vi "Periodic Tasks Curtis.vi"(8 "error in":errorcluster) -> ()   [LabVIEW 2016]
doc: "This VI runs in parallel to other tasks. It can contain as many user-defined periodic loops as you need. These can carry out PID or other sorts of timed response."
uses:
  <userlib>/836-libraries/Drive/Drive_Code/Drive_Code_Support/Drive_Code_PID_Bundle.ctl
  <vilib>/Platform/TimedLoop/XDataNode/timing_clust.ctl
  <vilib>/Platform/TimedLoop/XDataNode/nitl_modes.ctl
  <vilib>/Platform/TimedLoop/XDataNode/wakeup.ctl
  <vilib>/Rock Robotics/WPI/RobotDrive/WPI_RobotDriveDevRef.ctl
  <vilib>/Rock Robotics/WPI/MotorControl/WPI_MotorControlDeviceRef.ctl
  <vilib>/Rock Robotics/WPI/MotorControl/WPI_MotorControlType.ctl
  <vilib>/Rock Robotics/SystemInterfaces/DIO/FPGA_DIOPWMChannel.ctl
  <vilib>/Rock Robotics/WPI/PWM/WPI_PWMDeadband.ctl
  <vilib>/Rock Robotics/WPI/ThirdParty/CanMotor/TalonSRX/WPI_CANTalonSRX_APIControlMode.ctl
  <vilib>/Rock Robotics/WPI/Utilities/WPI_GetSetVariantRefNum.vi
  <vilib>/addons/control/pid/pid.llb/PID (DBL).vi
  <vilib>/platform/TimedLoop/XDataNode/XDataNode.xnode
  <vilib>/Platform/TimedLoop/XDataNode/XDNodeRunTimeDep.lvlib
  <vilib>/addons/control/pid/NI_PID_pid.lvlib
panel:
  in  "reset":bool
  in  "PID gains 2":T1={"proportional gain (Kc)"=0.025, "integral time (Ti, min)"=0.0, "derivative time (Td, min)"=0.01} {"derivative time (Td, min)" format="%.3f"; "integral time (Ti, min)" format="%.3f"; "proportional gain (Kc)" format="%.3f"}
  in  "Offset":dbl=20.0
  in  "Max Throttle":dbl=0.35
  in  "Negate":bool=TRUE
  in  "Follow Cam":bool=TRUE
  in  "PID Gains 2":T2={"Yaw, Driving Straight"={"proportional gain (Kc)"=0.08, "integral time (Ti, min)"=0.0, "derivative time (Td, min)"=0.0}, "Yaw, Holding Still"={"proportional gain (Kc)"=0.0, "integral time (Ti, min)"=0.0, "derivative time (Td, min)"=0.0}, "Distance, Driving Straight"={"proportional gain (Kc)"=0.0, "integral time (Ti, min)"=0.0, "derivative time (Td, min)"=0.0}, "Distance, Holding Still"={"proportional gain (Kc)"=0.0, "integral time (Ti, min)"=0.0, "derivative time (Td, min)"=0.0}}
  in  "reset":bool
  in  "PID Gains":T2
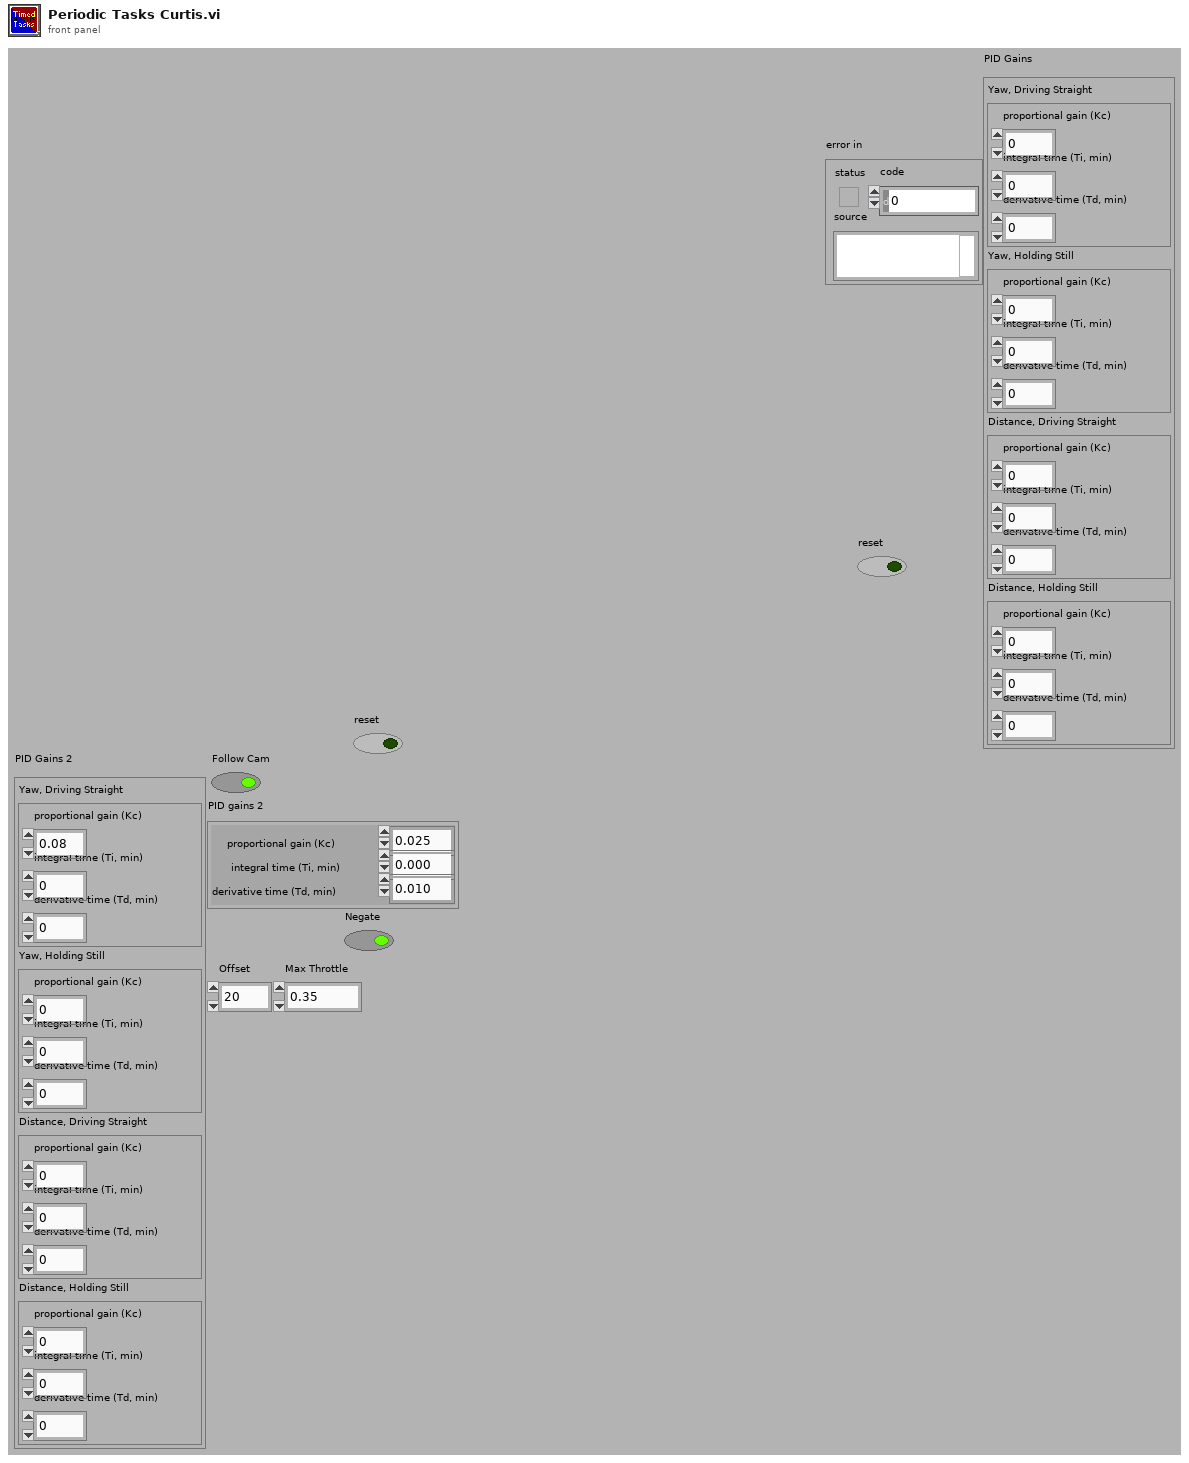
[diagram p1: front panel]
types:
  T1 = cluster{"proportional gain (Kc)":dbl, "integral time (Ti, min)":dbl, "derivative time (Td, min)":dbl}
  T2 = typedef "Drive_Code_PID_Bundle.ctl" = cluster{"Yaw, Driving Straight":cluster{"proportional gain (Kc)":dbl, "integral time (Ti, min)":dbl, "derivative time (Td, min)":dbl}, "Yaw, Holding Still":cluster{"proportional gain (Kc)":dbl, "integral time (Ti, min)":dbl, "derivative time (Td, min)":dbl}, "Distance, Driving Straight":cluster{"proportional gain (Kc)":dbl, "integral time (Ti, min)":dbl, "derivative time (Td, min)":dbl}, "Distance, Holding Still":cluster{"proportional gain (Kc)":dbl, "integral time (Ti, min)":dbl, "derivative time (Td, min)":dbl}}
  T3 = typedef "WPI_RobotDriveDevRef.ctl" = cluster{"DevStatus":errorcluster, "Motors[]":T4[], "Square Inputs":bool, "Max Output":dbl}
  T4 = typedef "WPI_MotorControlDeviceRef.ctl" = cluster{"DeviceStatus":errorcluster, "Type":T5, "PWM":cluster{"PWM Channel":T6, "DeadBand":T7}, "CAN":cluster{"Device Number":u8, "SetOutput VI Ref":variant, "GetOutput VI Ref":variant, "Enable VI Ref":variant, "Disable VI Ref":variant, "Data":variant}, "Invert":bool}
  T5 = typedef "WPI_MotorControlType.ctl" = enum16{"PWM", "CAN"}
  T6 = typedef "FPGA_DIOPWMChannel.ctl" = enum8{"PWM 0", "PWM 1", "PWM 2", "PWM 3", "PWM 4", "PWM 5", "PWM 6", "PWM 7", "PWM 8", "PWM 9", "PWM MXP 0", "PWM MXP 1", "PWM MXP 2", "PWM MXP 3", "PWM MXP 4", "PWM MXP 5", "PWM MXP 6", "PWM MXP 7", "PWM MXP 8", "PWM MXP 9", "Invalid"}
  T7 = typedef "WPI_PWMDeadband.ctl" = cluster{"Name":string, "maxPositivePwm":i32, "minPositivePwm":i32, "centerPwm":i32, "maxNegativePwm":i32, "minNegativePwm":i32, "angularRange":u16}
  T8 = typedef "WPI_JoystickDevRef.ctl" = cluster{"Device":T9}
  T9 = typedef "WPI_JoystickDeviceEnum.ctl" = enum16{"USB 0", "USB 1", "USB 2", "USB 3", "USB 4", "USB 5"}
  T10 = typedef "WPI_EncoderDevRef.ctl" = cluster{"DevStatus":errorcluster, "EncoderIndex":T11, "CounterIndex":T12, "DistancePerCount":dbl, "Decoding Type":T13}
  T11 = typedef "FPGA_EncoderIdx.ctl" = enum8{"Enc 0", "Enc 1", "Enc 2", "Enc 3", "Enc 4", "Enc 5", "Enc 6", "Enc 7", "Invalid"}
  T12 = typedef "FPGA_CounterCtrSystemIndex.ctl" = enum8{"Ctr 0", "Ctr 1", "Ctr 2", "Ctr 3", "Ctr 4", "Ctr 5", "Ctr 6", "Ctr 7", "Invalid"}
  T13 = typedef "WPI_EncoderType.ctl" = enum16{"1x", "2x", "4x"}
  T14 = cluster{"Yaw":dbl, "Roll":dbl, "Pitch":dbl, "Yaw Wind":dbl, "Roll Wind":dbl, "Pitch Wind":dbl}
  T15 = typedef "Drive_Code_Bundle.ctl" = cluster{"Sensor Data":T16, "Drive Command rt fifo":refnum<k33>, "Logging Data":refnum<k33>}
  T16 = typedef "Sensor_Cluster.ctl" = cluster{"Gyro Data":cluster{"Gyro RT FIFO":refnum<k33>, "Gyro Current":dbl, "Gyro Hold":dbl}, "Encoder Data":cluster{"Encoder RT FIFO":refnum<k33>, "Encoder Current":dbl, "Encoder Hold":dbl}, "Camera Data":cluster{"Camera RT FIFO":refnum<k33>, "Camera Current":T17}}
  T17 = typedef "Camera_Cluster.ctl" = cluster{" Angle":dbl, "Valid":bool}
  T18 = typedef "WPI_I2CDevRef.ctl" = cluster{"DevStatus":errorcluster, "Device Address":u8, "Handle":i32, "I2C Bus":T19}
  T19 = typedef "i2c_bus.ctl" = enum16{"I2C On-Board", "I2C MXP", "Invalid"}
  T20 = typedef "XDNodeRunTimeDep.lvlib/timing_clust.ctl" = cluster{"Expected End [f-1]":u64, "Actual End [f-1]":u64, "Finished Late? [f-1]":bool, "Expected End [i-1]":u64, "Actual End [i-1]":u64, "Finished Late? [i-1]":bool, "Expected Start [i]":u64, "Actual Start [i]":u64, "Expected Start [f]":u64, "Actual Start [f]":u64, "Source Name":string, "Structure Name":string, "Period":i64, "Deadline":i64, "Offset":i64, "Start":i64, "Priority":i32, "Timeout":i32, "Mode":T21, "Wakeup Reason":T22, "Error":errorcluster, "Source Type":string, "Secondary Source Type":string, "Global End Time":u64, "Global Start Time":u64, "Frame Duration":u64, "Iteration Duration":u64, "Assigned CPU":i32, "I/O Scan Engine Mode":u32}
  T21 = typedef "XDNodeRunTimeDep.lvlib/nitl_modes.ctl" = enum32{"No Change", "Process missed periods, maintain original phase", "Discard missed periods, maintain original phase", "Process missed periods, ignore original phase", "Discard missed periods, ignore original phase"}
  T22 = typedef "XDNodeRunTimeDep.lvlib/wakeup.ctl" = enum32{"Normal", "Aborted", "Asynchronous wakeup", "Timing source error", "Timed loop error", "Timeout"}
  T23 = typedef "WPI_CANTalonSRX_APIControlMode.ctl" = enum8{"Percent VBus", "Speed", "Position", "Slave", "Unchanged / Invalid", "Voltage Compensation", "Current", "Motion Profile", "Motion Magic"}
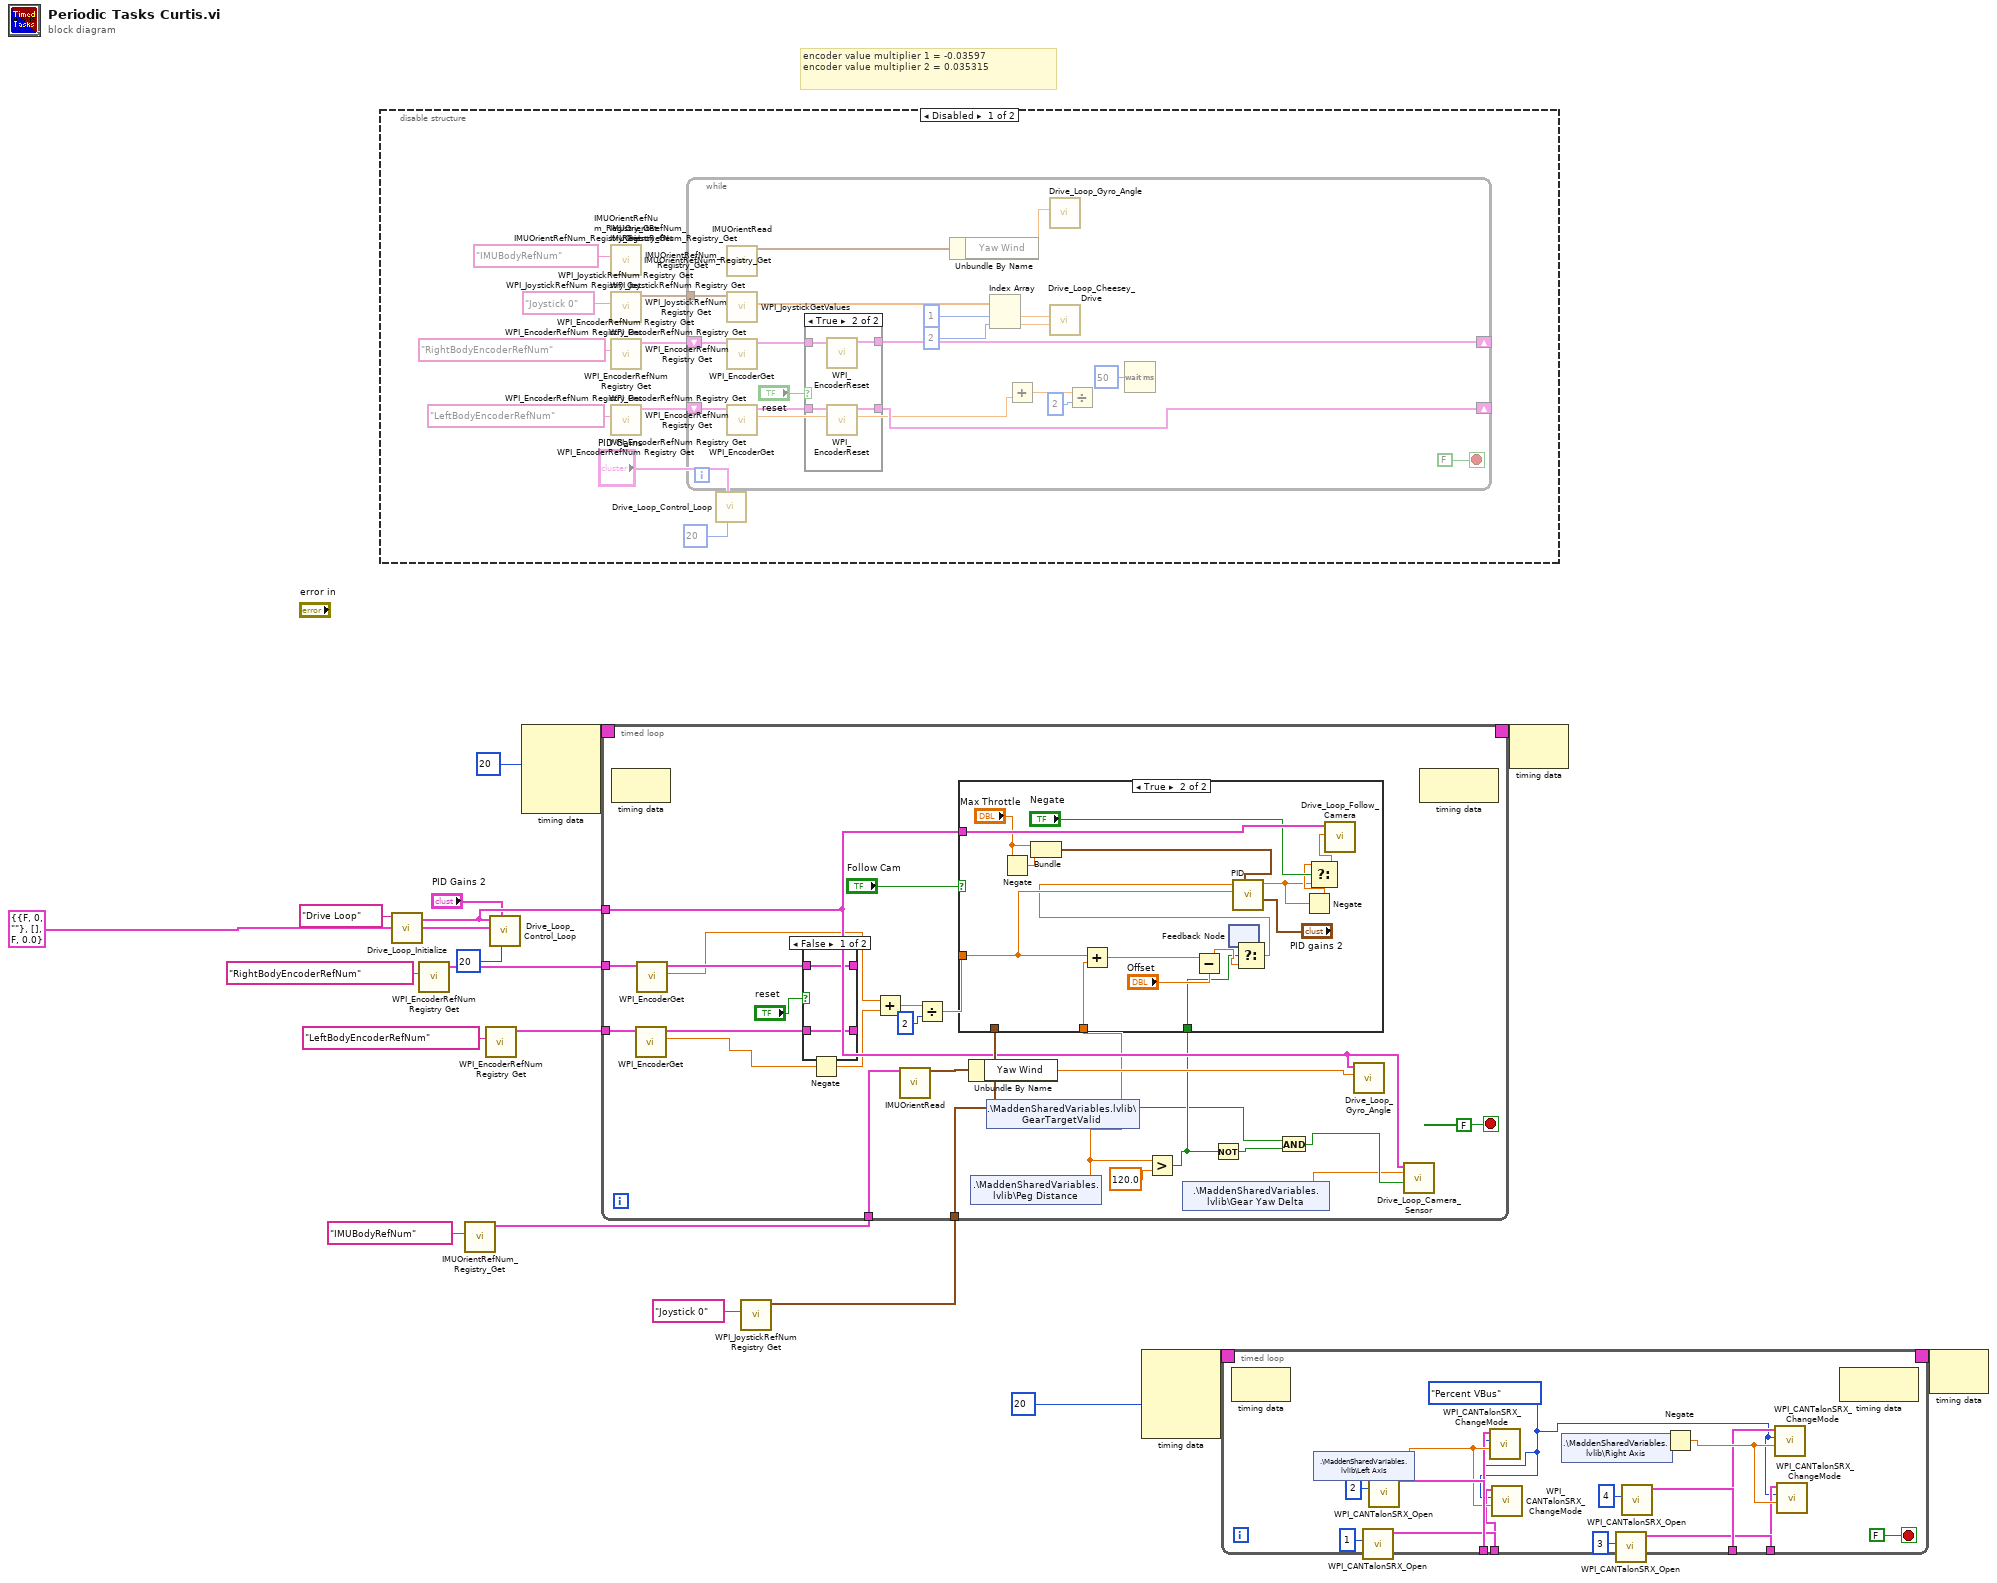
[diagram p0: block diagram]
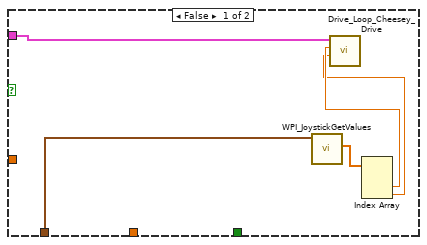
[diagram p2: hidden frame]
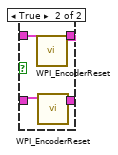
[diagram p3: hidden frame]
diagram:
  # "encoder value multiplier 1 = -0.03597\nencoder value multiplier 2 = 0.035315"
  n1 = disable-structure shown="Disabled" {
    frame Disabled {
      n2 = call <userlib>:"IMUOrientRefNum_Registry_Get.vi"("refnum name"="IMUBodyRefNum") -> ()  [unwired: 9 in, 2 out]
      n3 = call <userlib>:"IMUOrientRefNum_Registry_Get.vi"("refnum name"="IMUBodyRefNum") -> ()  [unwired: 9 in, 2 out]
      n4 = call <userlib>:"IMUOrientRefNum_Registry_Get.vi"("refnum name"="IMUBodyRefNum") -> ()  [unwired: 9 in, 2 out]
      n5 = call <userlib>:"IMUOrientRefNum_Registry_Get.vi"("refnum name"="IMUBodyRefNum") -> ()  [unwired: 9 in, 2 out]
      n6 = call <userlib>:"IMUOrientRefNum_Registry_Get.vi"("refnum name"="IMUBodyRefNum") -> ()  [unwired: 9 in, 2 out]
      n7 = call <userlib>:"IMUOrientRefNum_Registry_Get.vi"("refnum name"="IMUBodyRefNum") -> ()  [unwired: 9 in, 2 out]
      n8 = call <vilib>:"WPI_JoystickRefNum Registry Get.vi"("refnum name"="Joystick 0") -> ()  [unwired: 9 in, 2 out]
      n9 = call <vilib>:"WPI_JoystickRefNum Registry Get.vi"("refnum name"="Joystick 0") -> ()  [unwired: 9 in, 2 out]
      n10 = call <vilib>:"WPI_JoystickRefNum Registry Get.vi"("refnum name"="Joystick 0") -> ()  [unwired: 9 in, 2 out]
      n11 = call <vilib>:"WPI_JoystickRefNum Registry Get.vi"("refnum name"="Joystick 0") -> ("JoystickDevRef"=w44:T8)  [unwired: 9 in, 1 out]
      n12 = call <vilib>:"WPI_EncoderRefNum Registry Get.vi"("refnum name"="RightBodyEncoderRefNum") -> ()  [unwired: 9 in, 2 out]
      n13 = call <vilib>:"WPI_EncoderRefNum Registry Get.vi"("refnum name"="RightBodyEncoderRefNum") -> ()  [unwired: 9 in, 2 out]
      n14 = call <vilib>:"WPI_EncoderRefNum Registry Get.vi"("refnum name"="RightBodyEncoderRefNum") -> ()  [unwired: 9 in, 2 out]
      n15 = call <vilib>:"WPI_EncoderRefNum Registry Get.vi"("refnum name"="RightBodyEncoderRefNum") -> ()  [unwired: 9 in, 2 out]
      n16 = call <vilib>:"WPI_EncoderRefNum Registry Get.vi"("refnum name"="RightBodyEncoderRefNum") -> ("EncoderDevRef"=w47:T10)  [unwired: 9 in, 1 out]
      n17 = call <vilib>:"WPI_EncoderRefNum Registry Get.vi"("refnum name"="LeftBodyEncoderRefNum") -> ()  [unwired: 9 in, 2 out]
      n18 = call <vilib>:"WPI_EncoderRefNum Registry Get.vi"("refnum name"="LeftBodyEncoderRefNum") -> ()  [unwired: 9 in, 2 out]
      n19 = call <vilib>:"WPI_EncoderRefNum Registry Get.vi"("refnum name"="LeftBodyEncoderRefNum") -> ()  [unwired: 9 in, 2 out]
      n20 = call <vilib>:"WPI_EncoderRefNum Registry Get.vi"("refnum name"="LeftBodyEncoderRefNum") -> ()  [unwired: 9 in, 2 out]
      n21 = call <vilib>:"WPI_EncoderRefNum Registry Get.vi"("refnum name"="LeftBodyEncoderRefNum") -> ("EncoderDevRef"=w46:T10)  [unwired: 9 in, 1 out]
      n22 = while {
        tunnel: w44 -> [w66]
        shift-right: [w56] -> _
        shift-left: w47 -> [w73]
        shift-right: [w55] -> _
        shift-left: w46 -> [w72]
        stop <- FALSE stop-if-true
        n23 = call <userlib>:"IMUOrientRead.vi"() -> ("Orient Y/R/P"=w68:T14)  [unwired: 9 in, 6 out]
        n24 = call <vilib>:"WPI_JoystickGetValues.vi"("JoystickDevRef"=w66) -> ("Axes"=w65:dbl[])  [unwired: 6 in, 4 out]
        n25 = call <vilib>:"WPI_EncoderGet.vi"("EncoderDevRef"=w73) -> ("EncoderDevRef"=w58:T10)  [unwired: 5 in, 5 out]
        n26 = call <vilib>:"WPI_EncoderGet.vi"("EncoderDevRef"=w72) -> ("Distance"=w53:dbl, "EncoderDevRef"=w57:T10)  [unwired: 5 in, 4 out]
        n27 = case shown="True" "reset" {
          tunnel: w58 -> [w75 w79]
          tunnel: w57 -> [w74 w78]
          tunnel: [w75 w77] -> w56
          tunnel: [w74 w76] -> w55
          frame False {
          }
          frame True {
            n28 = call <vilib>:"WPI_EncoderReset.vi"("EncoderDevRef"=w79) -> ("EncoderDevRef"=w77:T10)  [unwired: 9 in, 1 out]
            n29 = call <vilib>:"WPI_EncoderReset.vi"("EncoderDevRef"=w78) -> ("EncoderDevRef"=w76:T10)  [unwired: 9 in, 1 out]
          }
        }
        n30 = Unbundle By Name(w68) -> ("Yaw Wind"=w67:dbl)
        n31 = Index Array(array=w65, index #1=1 ("index"), index #2=2 ("index")) -> (element #1=w63:dbl, element #2=w62:dbl)
        n32 = Add(y=w53) -> (x+y=w71:dbl)  [unwired: 1 in]
        n33 = call <userlib>:"Drive_Loop_Gyro_Angle.vi"("Yaw Wind"=w67) -> ()  [unwired: 11 in]
        n34 = call <userlib>:"Drive_Loop_Cheesey_Drive.vi"("Wheel"=w62, "Throttle"=w63) -> ()  [unwired: 10 in]
        n35 = Divide(x=w71, y=2) -> (x/y=w69:dbl)
        n36 = Wait (ms)(milliseconds to wait=u32 50) -> ()  [unwired: 1 out]
      }
      n37 = call <userlib>:"Drive_Loop_Control_Loop.vi"("Period \n- Amount of time between iterations of the timed control loop"=i64 20 ("Period \n- Amount of time between iterations of the timed control loop"), "PID Gains"="PID Gains") -> ()  [unwired: 10 in]
    }
    frame Enabled {
    }
  }
  n38 = call <userlib>:"Drive_Loop_Initialize.vi"("Name of drive loop (give it a name!)"="Drive Loop") -> ("Drive Loop Cluster"=w14:T15)  [unwired: 9 in, 1 out]
  n39 = call <vilib>:"WPI_EncoderRefNum Registry Get.vi"("refnum name"="RightBodyEncoderRefNum") -> ("EncoderDevRef"=w9:T10)  [unwired: 9 in, 1 out]
  n40 = call <userlib>:"IMUOrientRefNum_Registry_Get.vi"("refnum name"="IMUBodyRefNum") -> ("I2CDevRef out"=w12:T18)  [unwired: 9 in, 1 out]
  n41 = call <vilib>:"WPI_EncoderRefNum Registry Get.vi"("refnum name"="LeftBodyEncoderRefNum") -> ("EncoderDevRef"=w8:T10)  [unwired: 9 in, 1 out]
  n42 = call <userlib>:"Drive_Loop_Control_Loop.vi"("Period \n- Amount of time between iterations of the timed control loop"=i64 20 ("Period \n- Amount of time between iterations of the timed control loop"), "PID Gains"="PID Gains 2", "RobotDriveDevRef"=T3 {"DevStatus"={"status"=FALSE, "code"=0, "source"=""}, "Motors[]"=[], "Square Inputs"=FALSE, "Max Output"=0.0}, "Control Cluster"=w14) -> ()  [unwired: 8 in]
  n43 = node-c288(i64 20 ("Period")) -> (w16:T20)  [unwired: 3 in]
  n44 = call <vilib>:"WPI_JoystickRefNum Registry Get.vi"("refnum name"="Joystick 0") -> ("JoystickDevRef"=w10:T8)  [unwired: 9 in, 1 out]
  n45 = timed-loop {
    tunnel: w14 -> [w99]
    timing: w16 -> [_]
    timing-out: [_] -> w15
    tunnel: w12 -> [w102]
    tunnel: w10 -> [w100]
    tunnel: w9 -> [w98]
    tunnel: w8 -> [w97]
    stop <- FALSE stop-if-true
    n46 = node-c288() -> ()  [unwired: 1 in, 1 out]
    n47 = call <vilib>:"WPI_EncoderGet.vi"("EncoderDevRef"=w97) -> ("Distance"=w81:dbl, "EncoderDevRef"=w95:T10)  [unwired: 5 in, 4 out]
    n48 = call <vilib>:"WPI_EncoderGet.vi"("EncoderDevRef"=w98) -> ("Distance"=w82:dbl, "EncoderDevRef"=w96:T10)  [unwired: 5 in, 4 out]
    n49 = case shown="False" "reset" {
      tunnel: w96 -> [w128 w132]
      tunnel: w95 -> [w127 w129]
      tunnel: [w128 w131] -> _
      tunnel: [w127 w130] -> _
      frame False {
      }
      frame True {
        n50 = call <vilib>:"WPI_EncoderReset.vi"("EncoderDevRef"=w132) -> ("EncoderDevRef"=w131:T10)  [unwired: 9 in, 1 out]
        n51 = call <vilib>:"WPI_EncoderReset.vi"("EncoderDevRef"=w129) -> ("EncoderDevRef"=w130:T10)  [unwired: 9 in, 1 out]
      }
    }
    n52 = Negate(x=w81) -> (-x=w83:dbl)
    n53 = Add(x=w82, y=w83) -> (x+y=w92:dbl)
    n54 = call <userlib>:"IMUOrientRead.vi"("I2CDevRef"=w102) -> ("Orient Y/R/P"=w101:T14)  [unwired: 8 in, 6 out]
    n55 = Divide(x=w92, y=2) -> (x/y=w91:dbl)
    n56 = Unbundle By Name(w101) -> ("Yaw Wind"=w90:dbl)
    n57 = shared-variable ".\\MaddenSharedVariables.lvlib\\Peg Distance"() -> (w88:dbl)  [unwired: 1 in, 1 out]
    n58 = shared-variable ".\\MaddenSharedVariables.lvlib\\GearTargetValid"() -> (w85:bool)  [unwired: 1 in, 1 out]
    n59 = Greater?(x=w88, y=120.0) -> (0:w87:bool)
    n60 = case shown="True" "Follow Cam" {
      tunnel: w99 -> [w109 w126]
      tunnel: w100 -> [w108 _]
      tunnel: w91 -> [_ w116]
      tunnel: w88 -> [_ w111]
      tunnel: w87 -> [_ w110]
      frame False {
        n61 = call <vilib>:"WPI_JoystickGetValues.vi"("JoystickDevRef"=w108) -> ("Axes"=w107:dbl[])  [unwired: 6 in, 4 out]
        n62 = Index Array(array=w107) -> (element #2=w106:dbl, element #3=w105:dbl)  [unwired: 3 in, 1 out]
        n63 = call <userlib>:"Drive_Loop_Cheesey_Drive.vi"("Wheel"=w105, "Throttle"=w106, "Drive Loop Cluster"=w109) -> ()  [unwired: 9 in]
      }
      frame True {
        n64 = Negate(x="Max Throttle") -> (-x=w122:dbl)
        n65 = Bundle("Max Throttle"="Max Throttle", w122) -> (w121:cluster{"Max Throttle":dbl, dbl})  [unwired: 1 in]
        n66 = Add(x=w116, y=w111) -> (x+y=w124:dbl)
        n67 = Subtract(x=w124, y="Offset") -> (x-y=w114:dbl)
        n68 = feedback #1() -> (w113:dbl)  [unwired: 1 in]
        n69 = Select(t=w113, s=w110, f=w114) -> (s? t:f=w112:dbl)
        n70 = feedback-in #1(w112) -> ()
        n71 = call-poly <vilib>:"PID.vi"("output range"=w121, "PID gains"="PID gains 2", "process variable"=w116, "setpoint"=w112) -> ("output"=w118:dbl)  [unwired: 6 in, 1 out]
        n72 = Negate(x=w118) -> (-x=w119:dbl)
        n73 = Select(t=w119, s="Negate", f=w118) -> (s? t:f=w117:dbl)
        n74 = call <userlib>:"Drive_Loop_Follow_Camera.vi"("Power Level #6"=w117, "Drive Loop Cluster"=w126) -> ()  [unwired: 10 in]
      }
    }
    n75 = shared-variable ".\\MaddenSharedVariables.lvlib\\Gear Yaw Delta"() -> (w80:dbl)  [unwired: 1 in, 1 out]
    n76 = Not(x=w87) -> (.not. x?=w86:bool)
    n77 = And(x=w85, y=w86) -> (x .and. y?=w84:bool)
    n78 = call <userlib>:"Drive_Loop_Gyro_Angle.vi"("Yaw Wind"=w90, "Drive Loop Cluster"=w99) -> ()  [unwired: 10 in]
    n79 = call <userlib>:"Drive_Loop_Camera_Sensor.vi"("Stable?"=w84, "Camera Angle"=w80, "Drive Loop Cluster"=w99) -> ()  [unwired: 9 in]
    n80 = node-c288() -> ()  [unwired: 1 in, 1 out]
  }
  n81 = node-c288(i64 20 ("Period")) -> (w27:T20)  [unwired: 3 in]
  n82 = call <vilib>:"WPI_CANTalonSRX_Open.vi"("Device Number"=u8 1) -> ("CAN Talon SRX Ref"=w22:T4)  [unwired: 9 in, 1 out]
  n83 = call <vilib>:"WPI_CANTalonSRX_Open.vi"("Device Number"=u8 2) -> ("CAN Talon SRX Ref"=w23:T4)  [unwired: 9 in, 1 out]
  n84 = node-c288(w15) -> ()  [unwired: 1 out]
  n85 = call <vilib>:"WPI_CANTalonSRX_Open.vi"("Device Number"=u8 3) -> ("CAN Talon SRX Ref"=w24:T4)  [unwired: 9 in, 1 out]
  n86 = call <vilib>:"WPI_CANTalonSRX_Open.vi"("Device Number"=u8 4) -> ("CAN Talon SRX Ref"=w25:T4)  [unwired: 9 in, 1 out]
  n87 = timed-loop {
    timing: w27 -> [_]
    timing-out: [_] -> w26
    tunnel: w25 -> [w140]
    tunnel: w24 -> [w139]
    tunnel: w23 -> [w138]
    tunnel: w22 -> [w137]
    stop <- FALSE stop-if-true
    w136 = WPI_CANTalonSRX_APIControlMode."Percent VBus" ("Control Mode")
    n88 = node-c288() -> ()  [unwired: 1 in, 1 out]
    n89 = shared-variable ".\\MaddenSharedVariables.lvlib\\Left Axis"() -> (w142:dbl)  [unwired: 1 in, 1 out]
    n90 = call <vilib>:"WPI_CANTalonSRX_ChangeMode.vi"("Output"=w142, "Control Mode"=w136, "CAN Talon SRX Ref"=w138) -> ()  [unwired: 7 in, 2 out]
    n91 = call <vilib>:"WPI_CANTalonSRX_ChangeMode.vi"("Output"=w142, "Control Mode"=w136, "CAN Talon SRX Ref"=w137) -> ()  [unwired: 7 in, 2 out]
    n92 = shared-variable ".\\MaddenSharedVariables.lvlib\\Right Axis"() -> (w143:dbl)  [unwired: 1 in, 1 out]
    n93 = Negate(x=w143) -> (-x=w141:dbl)
    n94 = call <vilib>:"WPI_CANTalonSRX_ChangeMode.vi"("Output"=w141, "Control Mode"=w136, "CAN Talon SRX Ref"=w140) -> ()  [unwired: 7 in, 2 out]
    n95 = call <vilib>:"WPI_CANTalonSRX_ChangeMode.vi"("Output"=w141, "Control Mode"=w136, "CAN Talon SRX Ref"=w139) -> ()  [unwired: 7 in, 2 out]
    n96 = node-c288() -> ()  [unwired: 1 in, 1 out]
  }
  n97 = node-c288(w26) -> ()  [unwired: 1 out]
